vi "Auto Vision.vi"(6 "Image Size":i32[](array[numeric])=[0, 120], 7 "Max Coordinate":i32[](array[numeric])=[0, 90], 9 "Rotational Velocity":dbl=0.1, 10 "Linear Velocity":dbl=0.3, 11 "Follow Colour ON":bool=TRUE) -> (0 "Done":bool, 2 "Rotational Velocity_After":dbl, 3 "Translational Velocity_After":dbl)   [LabVIEW 2015]
uses:
  <vilib>/vision/NI_Vision_Development_Module.lvlib
panel:
  in  "Kd Rotational Velocity":dbl=0.01 step=0.001
  out "Vertical Axis":i32
  out "Horizontal Axis":i32
  in  "Kp Linear Velocity":dbl=0.0375 step=0.01
  in  "Kd Linear Velocity":dbl=0.008 step=0.001
  in  "Kp Rotational Velocity":dbl=0.3 step=0.01
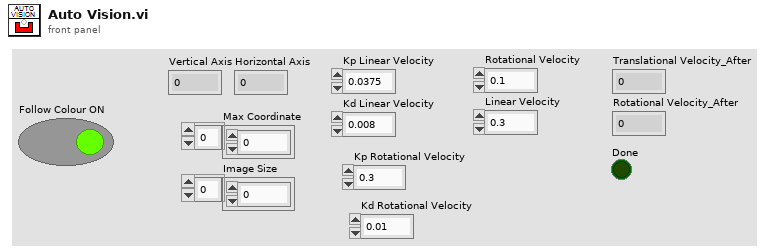
[diagram p1: front panel]
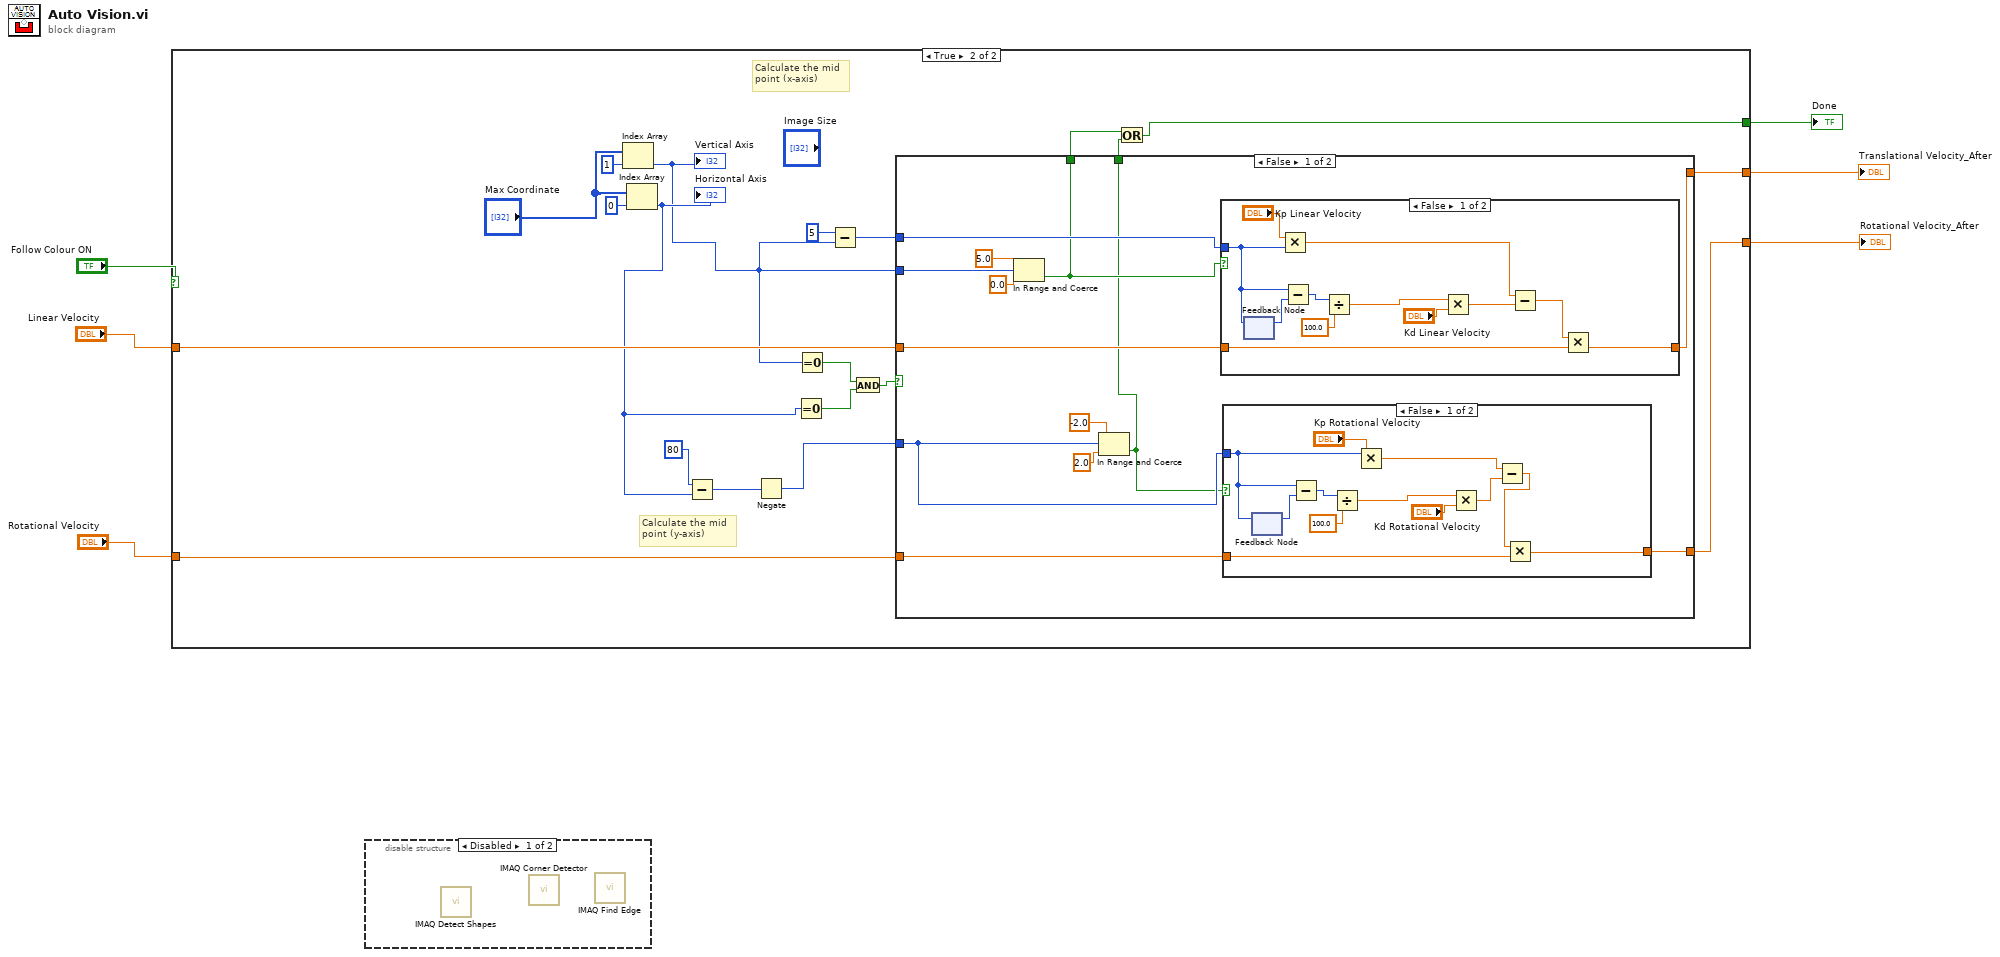
[diagram p0: block diagram]
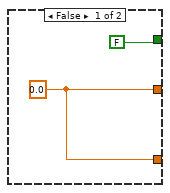
[diagram p3: hidden frame]
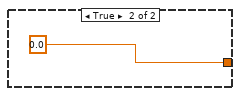
[diagram p4: hidden frame]
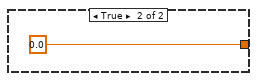
[diagram p5: hidden frame]
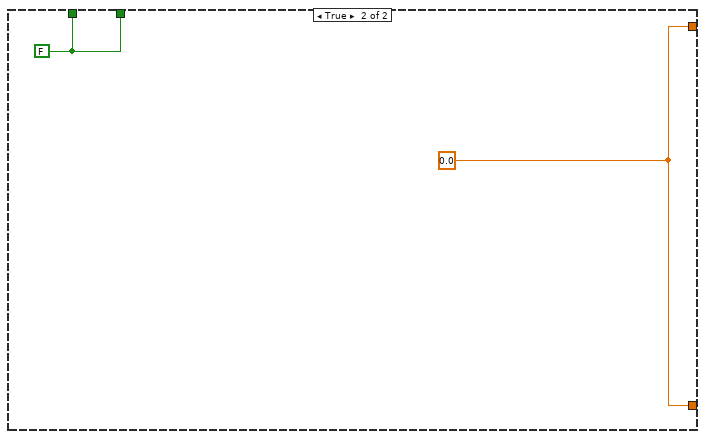
[diagram p6: hidden frame]
diagram:
  n1 = case shown="True" "Follow Colour ON" {
    tunnel: [w8 w26] -> w3
    tunnel: [w8 w25] -> w2
    tunnel: "Linear Velocity" -> [_ w28]
    tunnel: "Rotational Velocity" -> [_ w27]
    tunnel: [FALSE w9] -> w1
    frame False {
      w8 = 0.0
    }
    frame True {
      # "Calculate the mid\npoint (y-axis)"
      # "Calculate the mid\npoint (x-axis)"
      n2 = Index Array(array="Max Coordinate", index=1) -> (element=w14:i32)
      "Vertical Axis" <- w14
      n3 = Index Array(array="Max Coordinate", index=0) -> (element=w21:i32)
      "Horizontal Axis" <- w21
      n4 = Subtract(x=80 ("y"), y=w21) -> (x-y=w13:i32)
      n5 = Negate(x=w13) -> (-x=w12:i32)
      n6 = Equal To 0?(x=w21) -> (x = 0?=w19:bool)
      n7 = Equal To 0?(x=w14) -> (x = 0?=w20:bool)
      n8 = Subtract(x=5, y=w14) -> (x-y=w24:i32)
      n9 = And(x=w20, y=w19) -> (x .and. y?=w17:bool)
      n10 = case shown="False" w17 {
        tunnel: w28 -> [w41 _]
        tunnel: w27 -> [w40 _]
        tunnel: [w39 w69] -> w26
        tunnel: [w38 w69] -> w25
        tunnel: w12 -> [w35 _]
        tunnel: w24 -> [w32 _]
        tunnel: w14 -> [w31 _]
        tunnel: [w30 w68] -> w11
        tunnel: [w29 w68] -> w10
        frame False {
          n11 = In Range and Coerce(upper limit=5.0 ("y"), x=w31, lower limit=0.0 ("y")) -> (In Range?=w30:bool)  [unwired: 1 out]
          n12 = In Range and Coerce(upper limit=-2.0 ("lower limit"), x=w35, lower limit=2.0) -> (In Range?=w29:bool)  [unwired: 1 out]
          n13 = case shown="False" w30 {
            tunnel: w41 -> [w65 _]
            tunnel: [w66 0.0] -> w39
            tunnel: w32 -> [w62 _]
            frame False {
              n14 = feedback-in #1(w62) -> ()
              n15 = feedback #1() -> (w63:i32)  [unwired: 1 in]
              n16 = Multiply(x="Kp Linear Velocity", y=w62) -> (x*y=w56:dbl)
              n17 = Subtract(x=w62, y=w63) -> (x-y=w61:i32)
              n18 = Divide(x=w61, y=100.0) -> (x/y=w60:dbl)
              n19 = Multiply(x=w60, y="Kd Linear Velocity") -> (x*y=w58:dbl)
              n20 = Subtract(x=w56, y=w58) -> (x-y=w57:dbl)
              n21 = Multiply(x=w57, y=w65) -> (x*y=w66:dbl)
            }
            frame True {
            }
          }
          n22 = case shown="False" w29 {
            tunnel: w35 -> [w42 _]
            tunnel: w40 -> [w52 _]
            tunnel: [w51 0.0] -> w38
            frame False {
              n23 = feedback #2() -> (w46:i32)  [unwired: 1 in]
              n24 = feedback-in #2(w42) -> ()
              n25 = Subtract(x=w42, y=w46) -> (x-y=w47:i32)
              n26 = Divide(x=w47, y=100.0) -> (x/y=w48:dbl)
              n27 = Multiply(x=w42, y="Kp Rotational Velocity") -> (x*y=w45:dbl)
              n28 = Multiply(x=w48, y="Kd Rotational Velocity") -> (x*y=w44:dbl)
              n29 = Subtract(x=w45, y=w44) -> (x-y=w43:dbl)
              n30 = Multiply(x=w43, y=w52) -> (x*y=w51:dbl)
            }
            frame True {
            }
          }
        }
        frame True {
          w68 = FALSE
          w69 = 0.0
        }
      }
      n31 = Or(x=w11, y=w10) -> (x .or. y?=w9:bool)
    }
  }
  "Translational Velocity_After" <- w3
  "Rotational Velocity_After" <- w2
  "Done" <- w1
  n32 = disable-structure shown="Disabled" {
    frame Disabled {
      n33 = call-poly "IMAQ Detect Shapes"() -> ()  [unwired: 9 in, 3 out]
      n34 = call "IMAQ Corner Detector"() -> ()  [unwired: 10 in, 6 out]
      n35 = call "IMAQ Find Edge"() -> ()  [unwired: 8 in, 4 out]
    }
    frame Enabled {
    }
  }
